vi "房子數量.vi"(0 "房子 1":bool, 1 "房子 2":bool, 2 "房子 3":bool, 3 "房子 4":bool, 4 "旅館 1":bool, 5 "旅館 2":bool, 6 "旅館 3":bool, 7 "旅館 4":bool) -> (21 "房子數":dbl, 25 "旅館數":dbl)   [LabVIEW 2014]
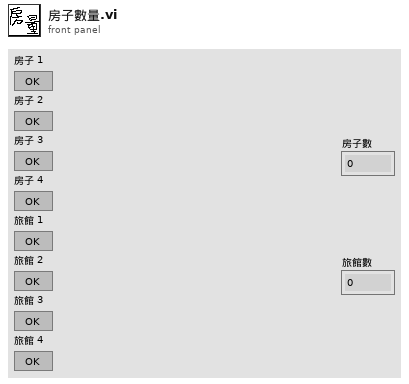
[diagram p1: front panel]
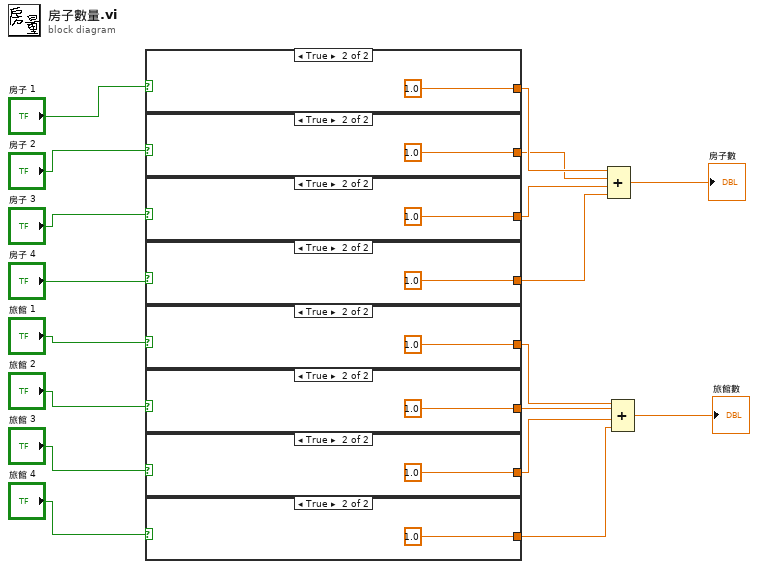
[diagram p0: block diagram]
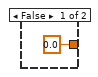
[diagram p2: hidden frame]
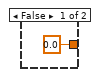
[diagram p3: hidden frame]
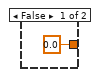
[diagram p4: hidden frame]
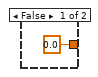
[diagram p5: hidden frame]
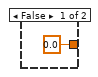
[diagram p6: hidden frame]
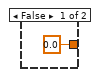
[diagram p7: hidden frame]
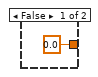
[diagram p8: hidden frame]
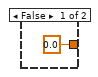
[diagram p9: hidden frame]
diagram:
  n1 = case shown="True" "房子 1" {
    tunnel: [0.0 1.0] -> w10
    frame False {
    }
    frame True {
    }
  }
  n2 = case shown="True" "房子 2" {
    tunnel: [0.0 1.0] -> w9
    frame False {
    }
    frame True {
    }
  }
  n3 = case shown="True" "房子 3" {
    tunnel: [0.0 1.0] -> w8
    frame False {
    }
    frame True {
    }
  }
  n4 = case shown="True" "房子 4" {
    tunnel: [0.0 1.0] -> w7
    frame False {
    }
    frame True {
    }
  }
  n5 = case shown="True" "旅館 1" {
    tunnel: [0.0 1.0] -> w6
    frame False {
    }
    frame True {
    }
  }
  n6 = case shown="True" "旅館 2" {
    tunnel: [0.0 1.0] -> w5
    frame False {
    }
    frame True {
    }
  }
  n7 = case shown="True" "旅館 3" {
    tunnel: [0.0 1.0] -> w4
    frame False {
    }
    frame True {
    }
  }
  n8 = case shown="True" "旅館 4" {
    tunnel: [0.0 1.0] -> w3
    frame False {
    }
    frame True {
    }
  }
  n9 = Compound Arithmetic op=ADD(w10, w9, w8, w7) -> (→"房子數":dbl)
  n10 = Compound Arithmetic op=ADD(w6, w5, w4, w3) -> (→"旅館數":dbl)
